vi "readProcessFlow.vi"(8 "error in (no error)":errorcluster, 10 "id":T1=1, 11 "CoolerControler in":refnum<class "CoolerControler.lvclass">) -> (0 "error out":errorcluster, 2 "flow":sgl, 3 "CoolerControler out":refnum<class "CoolerControler.lvclass">)   [LabVIEW 2016, in "CoolerControler.lvclass"]
uses:
  CoolerControler.lvclass
  typedefs/CoolerId.ctl
  SerialCommand/CoolerSerialCommand.lvclass
  typedefs/dataUnit.ctl
  typedefs/CoolerQuery.ctl
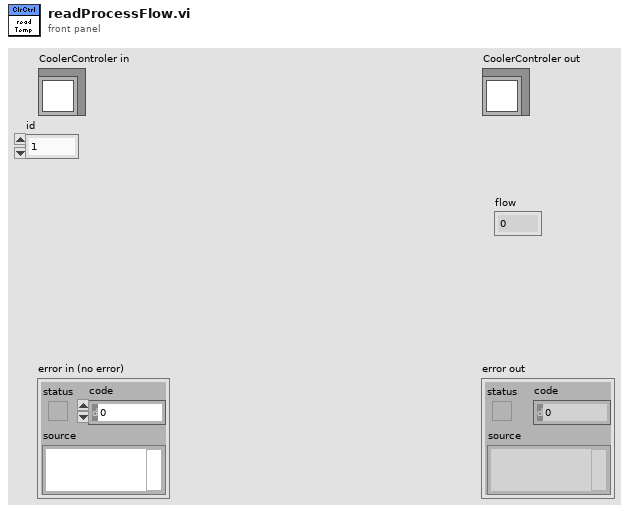
[diagram p1: front panel]
types:
  T1 = typedef "CoolerId.ctl" = u16
  T2 = typedef "CoolerQuery.ctl" = enum16{"ReadSerialWatchdog", "ReadControlSensor", "ReadSetTemperature", "ReadSupplyTemperature", "ReadExternalRTD", "ReadExternalThermistor", "ReadReturnTemperature", "ReadAmbientTemperature", "ReadProcessFlow", "ReadTECBank1Current", "ReadTECBank2Current", "ReadTEDriveLevel", "ReadAlarmStateLevel1", "ReadAlarmStateLevel21", "ReadAlarmStateLevel22", "ReadWarningStateLevel1", "ReadHighSupplyTempWarning", "ReadLowSupplyTempWarning", "ReadHighAmbientTempWarning", "ReadLowAmbientTempWarning", "ReadLowProcessFlowWarning", "ReadHighSupplyTempAlarm", "ReadLowSupplyTempAlarm", "ReadHighAmbientTempAlarm", "ReadLowAmbientTempAlarm", "ReadLowProcessFlowAlarm", "ReadPWMandRelayStatus", "ReadPIDStatus", "ReadUnitUpTime", "ReadFan1Speed", "ReadFan2Speed", "ReadFan3Speed", "ReadFan4Speed"}
  T3 = typedef "dataUnit.ctl" = enum16{"temperature", "flow", "current", "PID", "fanSpeed", "time", "PWM", "TEDriveLevel", "Number"}
  T4 = typedef "response.ctl" = cluster{"deviceId":string, "commandNumber":string, "errorActive":bool, "commandName":string, "responseData":string, "checkSum":string}
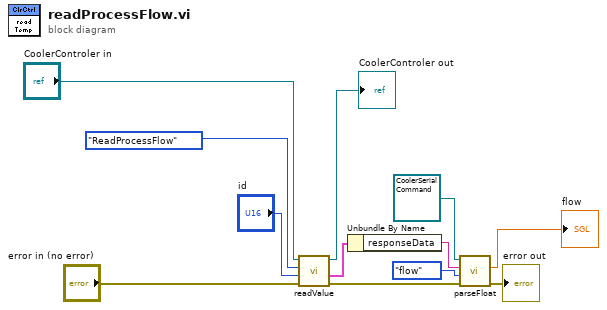
[diagram p0: block diagram]
diagram:
  n1 = call "readValue.vi"("error in (no error)"="error in (no error)", "id"="id", "CoolerQuery"=CoolerQuery."ReadProcessFlow", "CoolerControler in"="CoolerControler in") -> ("error out"=w5:errorcluster, "response out"=w7:T4, "CoolerControler out"=→"CoolerControler out":refnum<class "CoolerControler.lvclass">)  [unwired: 4 in, 1 out]
  n2 = Unbundle By Name(w7) -> ("responseData"=w6:string)
  n3 = call "parseFloat.vi"("error in (no error)"=w5, "unit"=dataUnit."flow", "commandData"=w6, "CoolerSerialCommand in"=refnum<class "CoolerSerialCommand.lvclass"> refnum) -> ("error out"=→"error out":errorcluster, "value"=→"flow":sgl)  [unwired: 4 in, 2 out]
